vi "Task Type.vi"(11 "SeqManager in":refnum<class "SeqManager.lvclass">) -> (2 "Task Type":string)   [LabVIEW 2020, in "Volatus.lvlib" / "SeqManager.lvclass"]
uses:
  SeqManager.lvclass
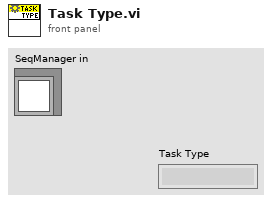
[diagram p1: front panel]
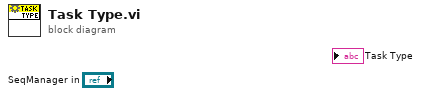
[diagram p0: block diagram]
diagram:
